vi "sub_handle_kf.vi"(8 "Pin":T1, 9 "Uin":dbl[](array[numeric]), 10 "Xin":dbl[](array[numeric]), 11 "Zin":dbl[](array[numeric])) -> (2 "Pout":T1, 3 "Xout":dbl[](array[numeric]))   [LabVIEW 2013]
uses:
  <vilib>/Analysis/Matrix/Datatypes/RealMatrix.ctl
  <vilib>/Analysis/baseanly.llb/A x Vector.vi
  <vilib>/Analysis/baseanly.llb/Real A x B.vi
  <vilib>/Analysis/_algsub.llb/Real PseudoInverse Matrix.vi
  <vilib>/Analysis/Matrix/Numeric/Subtract/Subtract - RM,RM.vi
  <vilib>/Analysis/Matrix/Numeric/Add/Add - RM,RM.vi
  <vilib>/Analysis/NI_AALBase.lvlib
  <vilib>/Analysis/Matrix/NI_Matrix.lvlib
  <vilib>/Analysis/NI_AALPro.lvlib
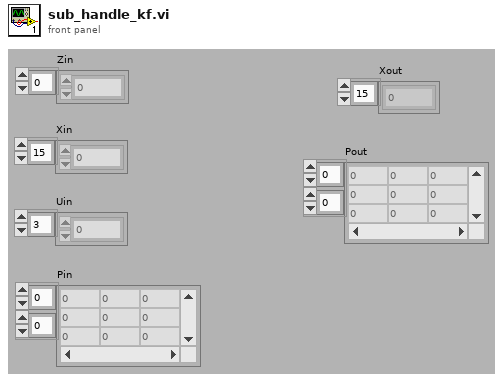
[diagram p1: front panel]
types:
  T1 = typedef "NI_Matrix.lvlib/RealMatrix.ctl" = dbl[][]
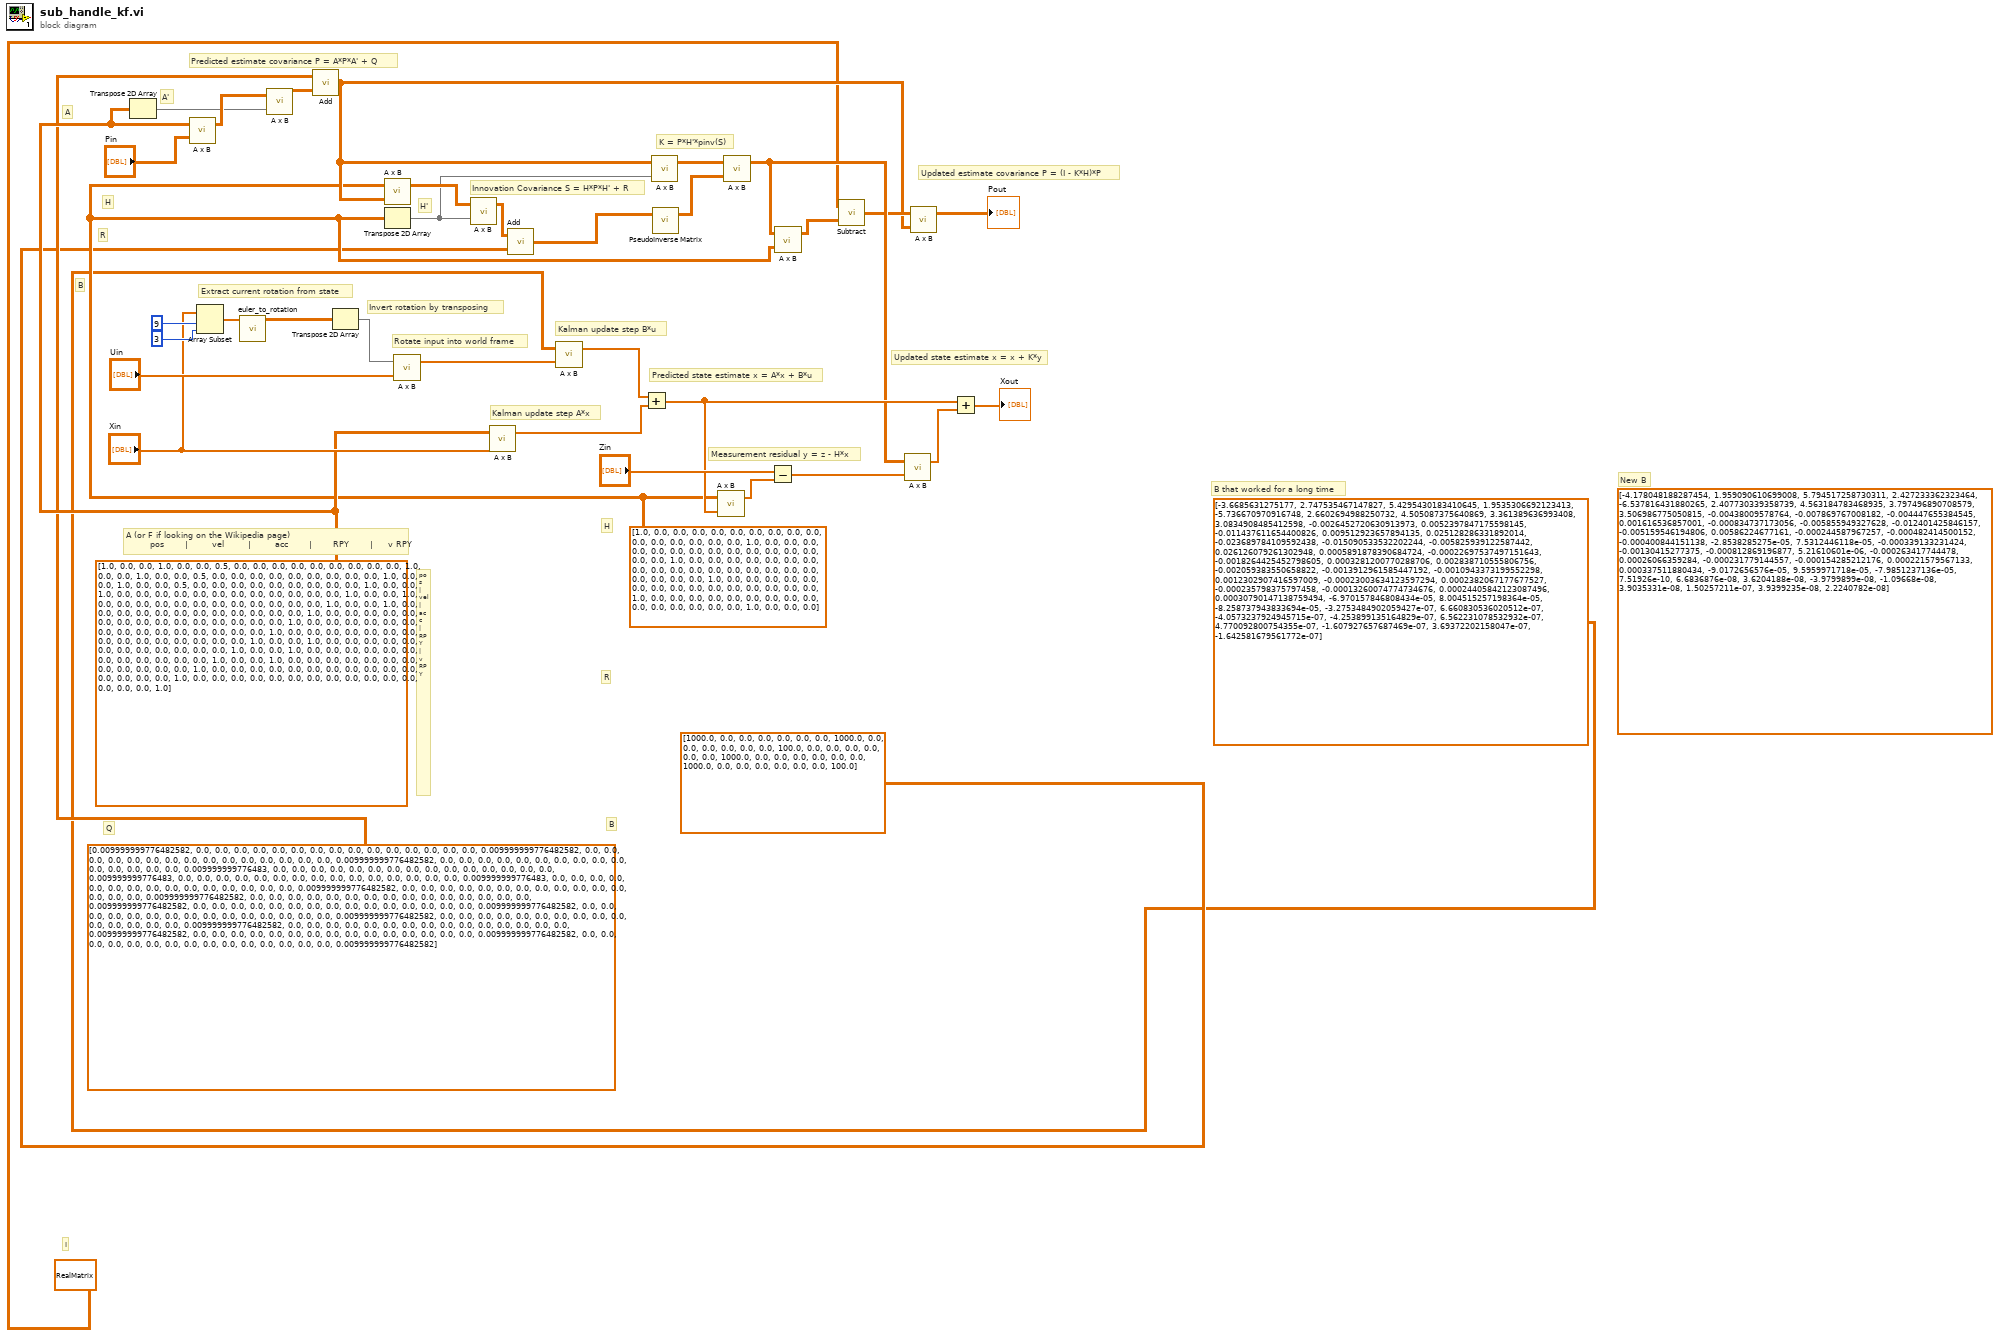
[diagram p0: block diagram]
diagram:
  (unwired) T1 [[-4.178048188287454, 1.959090610699008, 5.794517258730311], [2.427233362323464, -6.537816431880265, 2.407730339358739], [4.563184783468935, 3.797496890708579, 3.506986775050815], [-0.00438009578764, -0.007869767008182, -0.004447655384545], [0.001616536857001, -0.000834737173056, -0.005855949327628], [-0.012401425846157, -0.005159546194806, 0.00586224677161], [-0.000244587967257, -0.000482414500152, -0.000400844151138], [-2.8538285275e-05, 7.5312446118e-05, -0.000339133231424], [-0.00130415277375, -0.000812869196877, 5.21610601e-06], [-0.000263417744478, 0.00026066359284, -0.000231779144557], [-0.000154285212176, 0.000221579567133, 0.000337511880434], [-9.0172656576e-05, 9.5959971718e-05, -7.9851237136e-05], [7.51926e-10, 6.6836876e-08, 3.6204188e-08], [-3.9799899e-08, -1.09668e-08, 3.9035331e-08], [1.50257211e-07, 3.9399235e-08, 2.2240782e-08]] ("A + B")
  w7 = T1 [[1.0, 0.0, 0.0, 0.0, 0.0, 0.0, 0.0, 0.0, 0.0, 0.0, 0.0, 0.0, 0.0, 0.0, 0.0], [0.0, 1.0, 0.0, 0.0, 0.0, 0.0, 0.0, 0.0, 0.0, 0.0, 0.0, 0.0, 0.0, 0.0, 0.0], [0.0, 0.0, 1.0, 0.0, 0.0, 0.0, 0.0, 0.0, 0.0, 0.0, 0.0, 0.0, 0.0, 0.0, 0.0], [0.0, 0.0, 0.0, 0.0, 0.0, 0.0, 0.0, 0.0, 0.0, 1.0, 0.0, 0.0, 0.0, 0.0, 0.0], [0.0, 0.0, 0.0, 0.0, 0.0, 0.0, 0.0, 0.0, 0.0, 0.0, 1.0, 0.0, 0.0, 0.0, 0.0], [0.0, 0.0, 0.0, 0.0, 0.0, 0.0, 0.0, 0.0, 0.0, 0.0, 0.0, 1.0, 0.0, 0.0, 0.0]] ("A + B")
  w8 = T1 [[1.0, 0.0, 0.0, 1.0, 0.0, 0.0, 0.5, 0.0, 0.0, 0.0, 0.0, 0.0, 0.0, 0.0, 0.0], [0.0, 1.0, 0.0, 0.0, 1.0, 0.0, 0.0, 0.5, 0.0, 0.0, 0.0, 0.0, 0.0, 0.0, 0.0], [0.0, 0.0, 1.0, 0.0, 0.0, 1.0, 0.0, 0.0, 0.5, 0.0, 0.0, 0.0, 0.0, 0.0, 0.0], [0.0, 0.0, 0.0, 1.0, 0.0, 0.0, 1.0, 0.0, 0.0, 0.0, 0.0, 0.0, 0.0, 0.0, 0.0], [0.0, 0.0, 0.0, 0.0, 1.0, 0.0, 0.0, 1.0, 0.0, 0.0, 0.0, 0.0, 0.0, 0.0, 0.0], [0.0, 0.0, 0.0, 0.0, 0.0, 1.0, 0.0, 0.0, 1.0, 0.0, 0.0, 0.0, 0.0, 0.0, 0.0], [0.0, 0.0, 0.0, 0.0, 0.0, 0.0, 1.0, 0.0, 0.0, 0.0, 0.0, 0.0, 0.0, 0.0, 0.0], [0.0, 0.0, 0.0, 0.0, 0.0, 0.0, 0.0, 1.0, 0.0, 0.0, 0.0, 0.0, 0.0, 0.0, 0.0], [0.0, 0.0, 0.0, 0.0, 0.0, 0.0, 0.0, 0.0, 1.0, 0.0, 0.0, 0.0, 0.0, 0.0, 0.0], [0.0, 0.0, 0.0, 0.0, 0.0, 0.0, 0.0, 0.0, 0.0, 1.0, 0.0, 0.0, 1.0, 0.0, 0.0], [0.0, 0.0, 0.0, 0.0, 0.0, 0.0, 0.0, 0.0, 0.0, 0.0, 1.0, 0.0, 0.0, 1.0, 0.0], [0.0, 0.0, 0.0, 0.0, 0.0, 0.0, 0.0, 0.0, 0.0, 0.0, 0.0, 1.0, 0.0, 0.0, 1.0], [0.0, 0.0, 0.0, 0.0, 0.0, 0.0, 0.0, 0.0, 0.0, 0.0, 0.0, 0.0, 1.0, 0.0, 0.0], [0.0, 0.0, 0.0, 0.0, 0.0, 0.0, 0.0, 0.0, 0.0, 0.0, 0.0, 0.0, 0.0, 1.0, 0.0], [0.0, 0.0, 0.0, 0.0, 0.0, 0.0, 0.0, 0.0, 0.0, 0.0, 0.0, 0.0, 0.0, 0.0, 1.0]] ("A + B")
  # "pos     |      vel       |     acc       |     RPY      |    v RPY"
  # "New B"
  # "B that worked for a long time"
  # "Updated state estimate x = x + K*y"
  # "Updated estimate covariance P = (I - K*H)*P"
  # "A'"
  # "Invert rotation by transposing"
  # "Measurement residual y = z - H*x"
  # "K = P*H'*pinv(S)"
  # "H'"
  # "R"
  # "H"
  # "Innovation Covariance S = H*P*H' + R"
  # "Predicted estimate covariance P = A*P*A' + Q"
  # "B"
  # "A"
  # "Predicted state estimate x = A*x + B*u"
  # "Kalman update step B*u"
  # "Kalman update step A*x"
  # "Rotate input into world frame"
  # "I"
  # "B"
  # "H"
  # "A (or F if looking on the Wikipedia page)\n        pos       |        vel        |        acc       |       RPY       |     v RPY"
  # "Extract current rotation from state"
  # "R"
  # "Q"
  n1 = Transpose 2D Array(2D array=w8) -> (transposed array=w25:T1)
  n2 = call-poly <vilib>:"A x B.vi"("B"="Pin", "A"=w8) -> ("A x B"=w26:T1)  [unwired: 1 out]
  n3 = Array Subset(array="Xin", index=9, length=3) -> (w3:dbl[])
  n4 = call "euler_to_rotation.vi"("Theta XYZ"=w3) -> ("Rotation"=w2:T1)  [unwired: 10 in]
  n5 = call-poly <vilib>:"A x B.vi"("B"=w25, "A"=w26) -> ("A x B"=w30:T1)  [unwired: 1 out]
  n6 = call-poly <vilib>:"Add.vi"("Real Matrix B"=w30, "Real Matrix A"=T1 [[0.009999999776482582, 0.0, 0.0, 0.0, 0.0, 0.0, 0.0, 0.0, 0.0, 0.0, 0.0, 0.0, 0.0, 0.0, 0.0], [0.0, 0.009999999776482582, 0.0, 0.0, 0.0, 0.0, 0.0, 0.0, 0.0, 0.0, 0.0, 0.0, 0.0, 0.0, 0.0], [0.0, 0.0, 0.009999999776482582, 0.0, 0.0, 0.0, 0.0, 0.0, 0.0, 0.0, 0.0, 0.0, 0.0, 0.0, 0.0], [0.0, 0.0, 0.0, 0.009999999776483, 0.0, 0.0, 0.0, 0.0, 0.0, 0.0, 0.0, 0.0, 0.0, 0.0, 0.0], [0.0, 0.0, 0.0, 0.0, 0.009999999776483, 0.0, 0.0, 0.0, 0.0, 0.0, 0.0, 0.0, 0.0, 0.0, 0.0], [0.0, 0.0, 0.0, 0.0, 0.0, 0.009999999776483, 0.0, 0.0, 0.0, 0.0, 0.0, 0.0, 0.0, 0.0, 0.0], [0.0, 0.0, 0.0, 0.0, 0.0, 0.0, 0.009999999776482582, 0.0, 0.0, 0.0, 0.0, 0.0, 0.0, 0.0, 0.0], [0.0, 0.0, 0.0, 0.0, 0.0, 0.0, 0.0, 0.009999999776482582, 0.0, 0.0, 0.0, 0.0, 0.0, 0.0, 0.0], [0.0, 0.0, 0.0, 0.0, 0.0, 0.0, 0.0, 0.0, 0.009999999776482582, 0.0, 0.0, 0.0, 0.0, 0.0, 0.0], [0.0, 0.0, 0.0, 0.0, 0.0, 0.0, 0.0, 0.0, 0.0, 0.009999999776482582, 0.0, 0.0, 0.0, 0.0, 0.0], [0.0, 0.0, 0.0, 0.0, 0.0, 0.0, 0.0, 0.0, 0.0, 0.0, 0.009999999776482582, 0.0, 0.0, 0.0, 0.0], [0.0, 0.0, 0.0, 0.0, 0.0, 0.0, 0.0, 0.0, 0.0, 0.0, 0.0, 0.009999999776482582, 0.0, 0.0, 0.0], [0.0, 0.0, 0.0, 0.0, 0.0, 0.0, 0.0, 0.0, 0.0, 0.0, 0.0, 0.0, 0.009999999776482582, 0.0, 0.0], [0.0, 0.0, 0.0, 0.0, 0.0, 0.0, 0.0, 0.0, 0.0, 0.0, 0.0, 0.0, 0.0, 0.009999999776482582, 0.0], [0.0, 0.0, 0.0, 0.0, 0.0, 0.0, 0.0, 0.0, 0.0, 0.0, 0.0, 0.0, 0.0, 0.0, 0.009999999776482582]] ("A + B")) -> ("A + B"=w11:T1)
  n7 = Transpose 2D Array(2D array=w2) -> (transposed array=w34:T1)
  n8 = call-poly <vilib>:"A x B.vi"("B"=w11, "A"=w7) -> ("A x B"=w24:T1)  [unwired: 1 out]
  n9 = Transpose 2D Array(2D array=w7) -> (transposed array=w14:T1)
  n10 = call-poly <vilib>:"A x B.vi"("Vector"="Uin", "A"=w34) -> ("A x Vector"=w33:dbl[])  [unwired: 1 out]
  n11 = call-poly <vilib>:"A x B.vi"("B"=w14, "A"=w24) -> ("A x B"=w23:T1)  [unwired: 1 out]
  n12 = call-poly <vilib>:"A x B.vi"("Vector"="Xin", "A"=w8) -> ("A x Vector"=w31:dbl[])  [unwired: 1 out]
  n13 = call-poly <vilib>:"Add.vi"("Real Matrix B"=T1 [[1000.0, 0.0, 0.0, 0.0, 0.0, 0.0], [0.0, 1000.0, 0.0, 0.0, 0.0, 0.0], [0.0, 0.0, 100.0, 0.0, 0.0, 0.0], [0.0, 0.0, 0.0, 1000.0, 0.0, 0.0], [0.0, 0.0, 0.0, 0.0, 1000.0, 0.0], [0.0, 0.0, 0.0, 0.0, 0.0, 100.0]] ("A + B"), "Real Matrix A"=w23) -> ("A + B"=w20:T1)
  n14 = call-poly <vilib>:"A x B.vi"("Vector"=w33, "A"=T1 [[-3.6685631275177, 2.747535467147827, 5.4295430183410645], [1.9535306692123413, -5.736670970916748, 2.6602694988250732], [4.505087375640869, 3.361389636993408, 3.0834908485412598], [-0.0026452720630913973, 0.0052397847175598145, -0.011437611654400826], [0.009512923657894135, 0.025128286331892014, -0.023689784109592438], [-0.015090533532202244, -0.005825939122587442, 0.026126079261302948], [0.0005891878390684724, -0.00022697537497151643, -0.0018264425452798605], [0.0003281200770288706, 0.002838710555806756, -0.002059383550658822], [-0.0013912961585447192, -0.0010943373199552298, 0.0012302907416597009], [-0.00023003634123597294, 0.0002382067177677527, -0.000235798375797458], [-0.00013260074774734676, 0.00024405842123087496, 0.00030790147138759494], [-6.970157846808434e-05, 8.004515257198364e-05, -8.258737943833694e-05], [-3.2753484902059427e-07, 6.660830536020512e-07, -4.0573237924945715e-07], [-4.253899135164829e-07, 6.562231078532932e-07, 4.770092800754355e-07], [-1.607927657687469e-07, 3.69372202158047e-07, -1.642581679561772e-07]] ("A + B")) -> ("A x Vector"=w32:dbl[])  [unwired: 1 out]
  n15 = Add(x=w32, y=w31) -> (x+y=w18:dbl[])
  n16 = call-poly <vilib>:"A x B.vi"("B"=w14, "A"=w11) -> ("A x B"=w21:T1)  [unwired: 1 out]
  n17 = call-poly <vilib>:"PseudoInverse Matrix.vi"("Input Matrix"=w20) -> ("PseudoInverse Matrix"=w19:T1)  [unwired: 1 in, 1 out]
  n18 = call-poly <vilib>:"A x B.vi"("Vector"=w18, "A"=w7) -> ("A x Vector"=w27:dbl[])  [unwired: 1 out]
  n19 = call-poly <vilib>:"A x B.vi"("B"=w19, "A"=w21) -> ("A x B"=w15:T1)  [unwired: 1 out]
  n20 = Subtract ("Subtract.vi")(x="Zin", y=w27) -> (x-y=w17:dbl[])
  n21 = call-poly <vilib>:"A x B.vi"("B"=w7, "A"=w15) -> ("A x B"=w13:T1)  [unwired: 1 out]
  n22 = call-poly <vilib>:"Subtract.vi"("Real Matrix B"=w13, "Real Matrix A"=T1 [[1.0, 0.0, 0.0, 0.0, 0.0, 0.0, 0.0, 0.0, 0.0, 0.0, 0.0, 0.0, 0.0, 0.0, 0.0], [0.0, 1.0, 0.0, 0.0, 0.0, 0.0, 0.0, 0.0, 0.0, 0.0, 0.0, 0.0, 0.0, 0.0, 0.0], [0.0, 0.0, 1.0, 0.0, 0.0, 0.0, 0.0, 0.0, 0.0, 0.0, 0.0, 0.0, 0.0, 0.0, 0.0], [0.0, 0.0, 0.0, 1.0, 0.0, 0.0, 0.0, 0.0, 0.0, 0.0, 0.0, 0.0, 0.0, 0.0, 0.0], [0.0, 0.0, 0.0, 0.0, 1.0, 0.0, 0.0, 0.0, 0.0, 0.0, 0.0, 0.0, 0.0, 0.0, 0.0], [0.0, 0.0, 0.0, 0.0, 0.0, 1.0, 0.0, 0.0, 0.0, 0.0, 0.0, 0.0, 0.0, 0.0, 0.0], [0.0, 0.0, 0.0, 0.0, 0.0, 0.0, 1.0, 0.0, 0.0, 0.0, 0.0, 0.0, 0.0, 0.0, 0.0], [0.0, 0.0, 0.0, 0.0, 0.0, 0.0, 0.0, 1.0, 0.0, 0.0, 0.0, 0.0, 0.0, 0.0, 0.0], [0.0, 0.0, 0.0, 0.0, 0.0, 0.0, 0.0, 0.0, 1.0, 0.0, 0.0, 0.0, 0.0, 0.0, 0.0], [0.0, 0.0, 0.0, 0.0, 0.0, 0.0, 0.0, 0.0, 0.0, 1.0, 0.0, 0.0, 0.0, 0.0, 0.0], [0.0, 0.0, 0.0, 0.0, 0.0, 0.0, 0.0, 0.0, 0.0, 0.0, 1.0, 0.0, 0.0, 0.0, 0.0], [0.0, 0.0, 0.0, 0.0, 0.0, 0.0, 0.0, 0.0, 0.0, 0.0, 0.0, 1.0, 0.0, 0.0, 0.0], [0.0, 0.0, 0.0, 0.0, 0.0, 0.0, 0.0, 0.0, 0.0, 0.0, 0.0, 0.0, 1.0, 0.0, 0.0], [0.0, 0.0, 0.0, 0.0, 0.0, 0.0, 0.0, 0.0, 0.0, 0.0, 0.0, 0.0, 0.0, 1.0, 0.0], [0.0, 0.0, 0.0, 0.0, 0.0, 0.0, 0.0, 0.0, 0.0, 0.0, 0.0, 0.0, 0.0, 0.0, 1.0]] ("A + B")) -> ("A - B"=w12:T1)
  n23 = call-poly <vilib>:"A x B.vi"("Vector"=w17, "A"=w15) -> ("A x Vector"=w16:dbl[])  [unwired: 1 out]
  n24 = call-poly <vilib>:"A x B.vi"("B"=w11, "A"=w12) -> ("A x B"=→"Pout":T1)  [unwired: 1 out]
  n25 = Add(x=w18, y=w16) -> (x+y=→"Xout":dbl[])
